vi "Compute Phase.vi"(6 "Main Clock Line (s)":dbl, 11 "GRF":dbl) -> (0 "HS":bool, 3 "Phase":dbl)   [LabVIEW 2018]
uses:
  Gait Phase Estimation/COBRA Gait Phase Estimation Library.lvlib
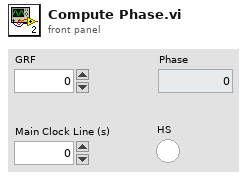
[diagram p1: front panel]
types:
  T1 = cluster{"Saturation Threshold":dbl, "LP Filter Cutoff\nFrequency":dbl, "HS Force Rate Threshold":dbl, "Sampling Frequency (Hz)":dbl, "Wait Window (s)":dbl}
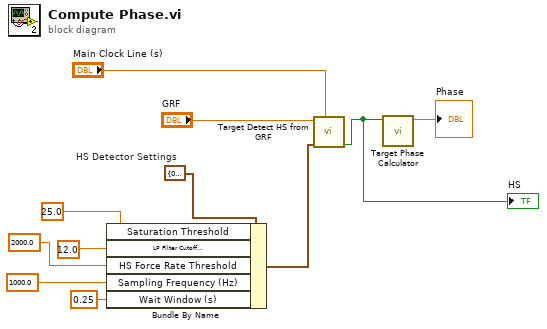
[diagram p0: block diagram]
diagram:
  w8 = T1 {"Saturation Threshold"=0.0, "LP Filter Cutoff\nFrequency"=12.0, "HS Force Rate Threshold"=0.0, "Sampling Frequency (Hz)"=0.0, "Wait Window (s)"=0.0}  # HS Detector Settings
  n1 = Bundle By Name(cluster=w8, "Saturation Threshold"=25.0, "LP Filter Cutoff\nFrequency"=12.0 ("LP Filter Cutoff\nFrequency"), "HS Force Rate Threshold"=2000.0 ("Sampling Frequency (Hz)"), "Sampling Frequency (Hz)"=1000.0 ("HS Threshold"), "Wait Window (s)"=0.25) -> (w2:T1)
  n2 = call "Target Detect HS from GRF.vi"("Main Clock Line (s)"="Main Clock Line (s)", "HS Detector Settings"=w2, "Fz"="GRF") -> ("HS"=w9:bool)  [unwired: 6 in, 2 out]
  "HS" <- w9
  n3 = call "Target Phase Calculator.vi"("HS Detected"=w9) -> ("Phase"=→"Phase":dbl)  [unwired: 10 in]
